vi "Write Registry Configuration.vi"(10 "Registry Configuration":T1, 11 "ConfigurableActor in":refnum<class "ConfigurableActor.lvclass">) -> (3 "ConfigurableActor out":refnum<class "ConfigurableActor.lvclass">)   [LabVIEW 2014, in "ConfigurableActor.lvclass"]
uses:
  ConfigurableActor.lvclass
  <vilib>/LabVIEW Open Source Project/Unicity/UniqueName/Registry/RegistryConfiguration.ctl
  <vilib>/LabVIEW Open Source Project/Unicity/Delimiter/Delimiter.lvclass
  <vilib>/LabVIEW Open Source Project/Unicity/RandomStringGenerator/RandomStringGenerator.lvclass
  <vilib>/LabVIEW Open Source Project/Unicity/UniqueName/UniquenessCriteria/UniquenessCriteria.lvclass
  <vilib>/LabVIEW Open Source Project/Unicity/UniqueName/StringIncrement/StringIncrement.lvclass
  ConfigurableActor.lvclass/ConfigurableActor.ctl
  <vilib>/LabVIEW Open Source Project/Unicity/UniqueName/Registry/NameRegistry.lvclass
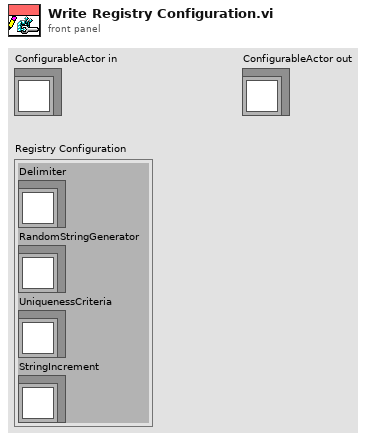
[diagram p1: front panel]
types:
  T1 = typedef "UniqueName.lvlib/NameRegistry.lvclass/RegistryConfiguration.ctl" = cluster{"Delimiter":refnum<class "Delimiter.lvclass">, "RandomStringGenerator":refnum<class "RandomStringGenerator.lvclass">, "UniquenessCriteria":refnum<class "UniquenessCriteria.lvclass">, "StringIncrement":refnum<class "StringIncrement.lvclass">}
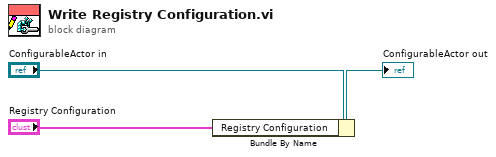
[diagram p0: block diagram]
diagram:
  n1 = Bundle By Name(cluster="ConfigurableActor in", "Registry Configuration"="Registry Configuration") -> (→"ConfigurableActor out":refnum<class "ConfigurableActor.lvclass">)
